vi "Priority.vi"(8 "error in (no error)":errorcluster, 11 "BadRequestException in":refnum<class "BadRequestException.lvclass">) -> (0 "error out":errorcluster, 2 "Priority":u16, 3 "BadRequestException out":refnum<class "BadRequestException.lvclass">)   [LabVIEW 2020, in "HTTP Server.lvlib" / "BadRequestException.lvclass"]
uses:
  BadRequestException.lvclass
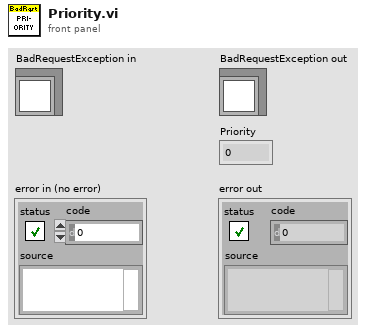
[diagram p1: front panel]
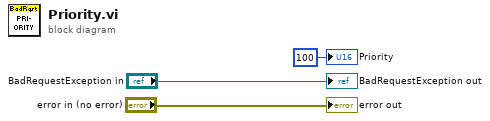
[diagram p0: block diagram]
diagram:
  "error out" <- "error in (no error)"
  "BadRequestException out" <- "BadRequestException in"
  "Priority" <- u16 100 ("Priority")
